vi "Check Logistic Square Pulse Midpoint Location.vi"(9 "Amplitude Array":dbl[](array[numeric]), 10 "t Array":dbl[](array[numeric]), 11 "Cursors in":dbl[](array[numeric])) -> (3 "Cursors out":dbl[](array[numeric]))   [LabVIEW 2021, in "Fits.lvlib"]
uses:
  Fits.lvlib
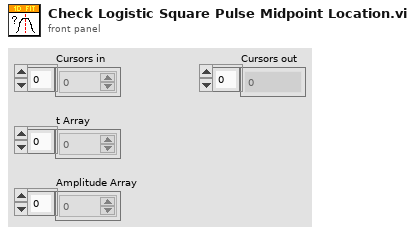
[diagram p1: front panel]
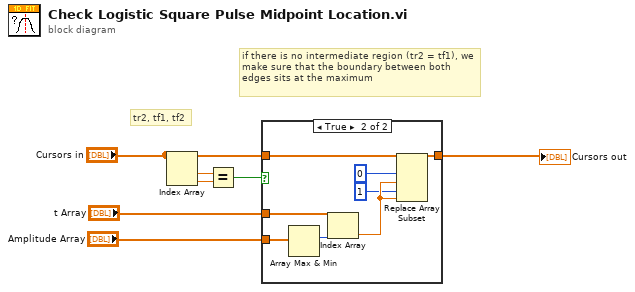
[diagram p0: block diagram]
diagram:
  # "if there is no intermediate region (tr2 = tf1), we make sure that the boundary between both edges sits at the maximum"
  # "tr2, tf1, tf2"
  n1 = Index Array(array="Cursors in") -> (element #1=w7:dbl, element #2=w6:dbl)  [unwired: 2 in]
  n2 = Equal?(x=w7, y=w6) -> (x = y?=w5:bool)
  n3 = case shown="True" w5 {
    tunnel: "Cursors in" -> [w8 w13]
    tunnel: [w8 w12] -> w3
    tunnel: "Amplitude Array" -> [_ w16]
    tunnel: "t Array" -> [_ w15]
    frame False {
    }
    frame True {
      n4 = Array Max & Min(array=w16) -> (max index (indices)=w14:i32)  [unwired: 3 out]
      n5 = Index Array(array=w15, index=w14) -> (element=w11:dbl)
      n6 = Replace Array Subset(array=w13, new element #1=w11, index #1=0 ("index"), new element #2=w11, index #2=1 ("index")) -> (w12:dbl[])
    }
  }
  "Cursors out" <- w3
